vi "Repeating Error Handler(RT).vi"   [LabVIEW 2017]
doc: "This merge VI includes additional structures needed to enable the \"retry\" option of the Specific Error Handler. See the Specific Error Handler VI for more information.\n\nThis VI is optimized for Real-Time applications. An alternate version for Windows VIs exists."
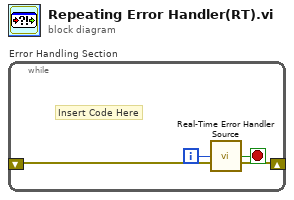
[diagram p0: block diagram]
diagram:
  n1 = while "Error Handling Section" {
    shift-right: [w3] -> _
    shift-left: _ -> [w4]
    i -> [w1]
    stop <- w2 stop-if-true
    # "Insert Code Here"
    n2 = call "Real-Time Error Handler Source"("Iteration"=w1, "Error to Check"=w4) -> ("Loop?"=w2:bool, "error out"=w3:errorcluster)  [unwired: 10 in, 2 out]
  }
